vi "Class Is Default Value.vi"(11 "Object":refnum<class>) -> (3 "Default Value":bool)   [LabVIEW 2020]
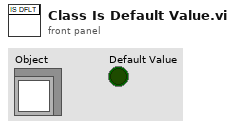
[diagram p1: front panel]
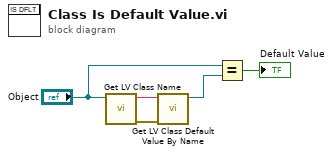
[diagram p0: block diagram]
diagram:
  n1 = call <vilib>:"Get LV Class Name.vi"("object"="Object") -> ("error out"=w5:errorcluster, "class name"=w4:string)  [unwired: 9 in]
  n2 = call <vilib>:"Get LV Class Default Value By Name.vi"("error in (no error)"=w5, "class name"=w4) -> ("object"=w3:refnum<class>)  [unwired: 8 in, 1 out]
  n3 = Equal?(x="Object", y=w3) -> (x = y?=→"Default Value":bool)
